vi "saveSettings.vi"(8 "error in (no error)":errorcluster, 10 "Path":path, 11 "PixelflySettings in":refnum<class "PixelflySettings.lvclass">) -> (0 "error out":errorcluster, 3 "PixelflySettings out":refnum<class "PixelflySettings.lvclass">)   [LabVIEW 2011, in "Tools.lvlib" / "Settings.lvlib" / "PixelflySettings.lvclass"]
uses:
  PixelflySettings.lvclass
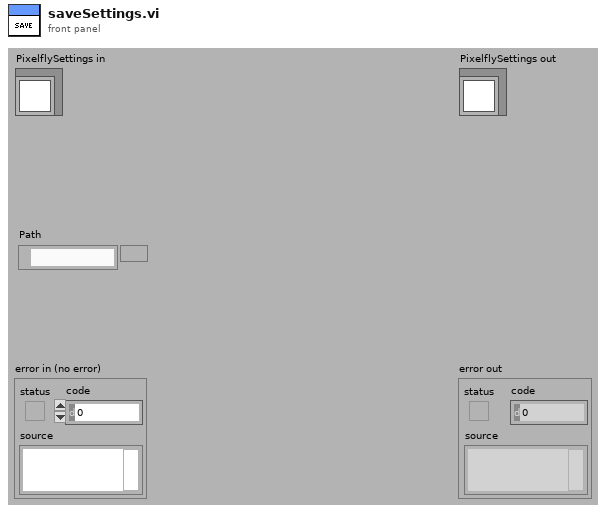
[diagram p1: front panel]
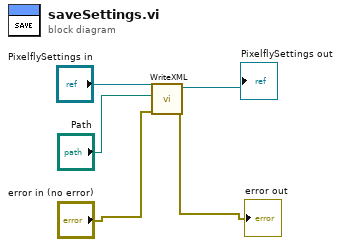
[diagram p0: block diagram]
diagram:
  n1 = call "WriteXML.vi"("error in (no error)"="error in (no error)", "Path"="Path", "PixelflySettings in"="PixelflySettings in") -> ("error out"=→"error out":errorcluster, "PixelflySettings out"=→"PixelflySettings out":refnum<class "PixelflySettings.lvclass">)  [unwired: 7 in]
